vi "Continuous Voltage Ouput - NI.vi"() -> ()   [LabVIEW 2022 SP3]
uses:
  WhiteNoise.ctl
  <vilib>/Utility/error.llb/DialogType.ctl
  <vilib>/DAQmx/write.llb/DAQmx Write (Analog 1D Wfm NChan NSamp).vi
  <vilib>/DAQmx/create/channels.llb/DAQmx Create Channel (AO-Voltage-Basic).vi
  <vilib>/DAQmx/configure/timing.llb/DAQmx Timing (Sample Clock).vi
  <vilib>/measure/maspectr.llb/FFT Spectrum (Mag-Phase) for N Chan.vi
  <vilib>/DAQmx/miscellaneous.llb/DAQmx Fill In Error Info.vi
  <resource>/objmgr/daqmx.rc
  <vilib>/measure/NI_MAPro.lvlib
  <vilib>/measure/NI_MABase.lvlib
panel:
  out "Mag":cluster{"f0":dbl, "df":dbl, "magnitude":dbl[]}[](graph)
  out "Phase":cluster{"f0":dbl, "df":dbl, "phase":dbl[]}[](graph)
  in  "Number of Samples":i32=40000
  in  "Sample Rate":dbl=41200.0
  in  "Sample Clock Source":tag="OnboardClock"
  in  "Max Voltage":dbl=3.5
  in  "Min Voltage":dbl=-3.0
  in  "Physical Channel(s)":tag="Dev1/ao0"
  in  "?":enum32{"White Noise", "Harmonic"}(tab)
  in  "Cluster":T2={"Seed"=0.0, "Standard Deviation"=0.2, "Reset"=FALSE, "Iterator"=1.0} {"Standard Deviation" format="%0.2p"}
  in  "Cluster 2":T3={"Iterator"=1.0, "Waveform Type"=0, "Frequency"=10.0, "Amplitude"=0.5} {"Frequency" format="%0.2p"; "Waveform Type" items=["Sine Wave", "Triangle Wave", "Square Wave", "Sawtooth Wave"]; "Amplitude" format="%0.2p"}
  out "Actual Sample Rate":dbl=1000.0 format="%0.2f"
  in  "Stop":bool
  out "Waveform Graph":waveform(dbl)[](graph)=[{"t0"=timestamp(0 s since 1904-01-01), "dt"=0.001, "Y"=[]}]
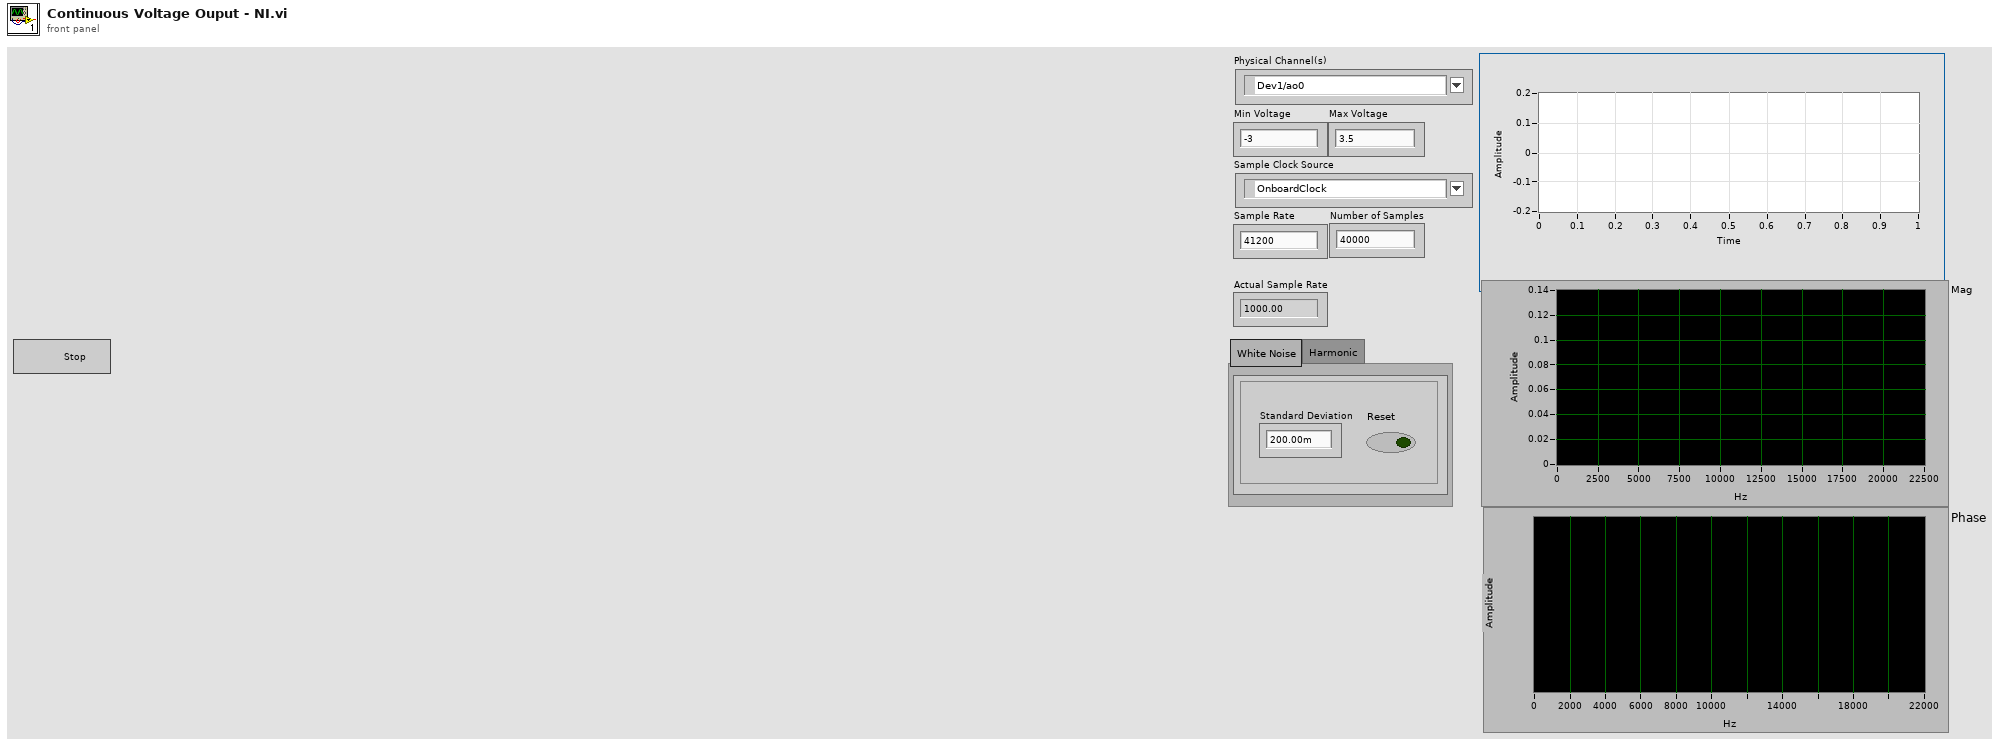
[diagram p1: front panel]
types:
  T1 = typedef "WhiteNoise.ctl" = dbl
  T2 = cluster{"Seed":T1, "Standard Deviation":dbl, "Reset":bool, "Iterator":dbl}
  T3 = cluster{"Iterator":dbl, "Waveform Type":u16, "Frequency":dbl, "Amplitude":dbl}
  T4 = typedef "DialogType.ctl" = u16
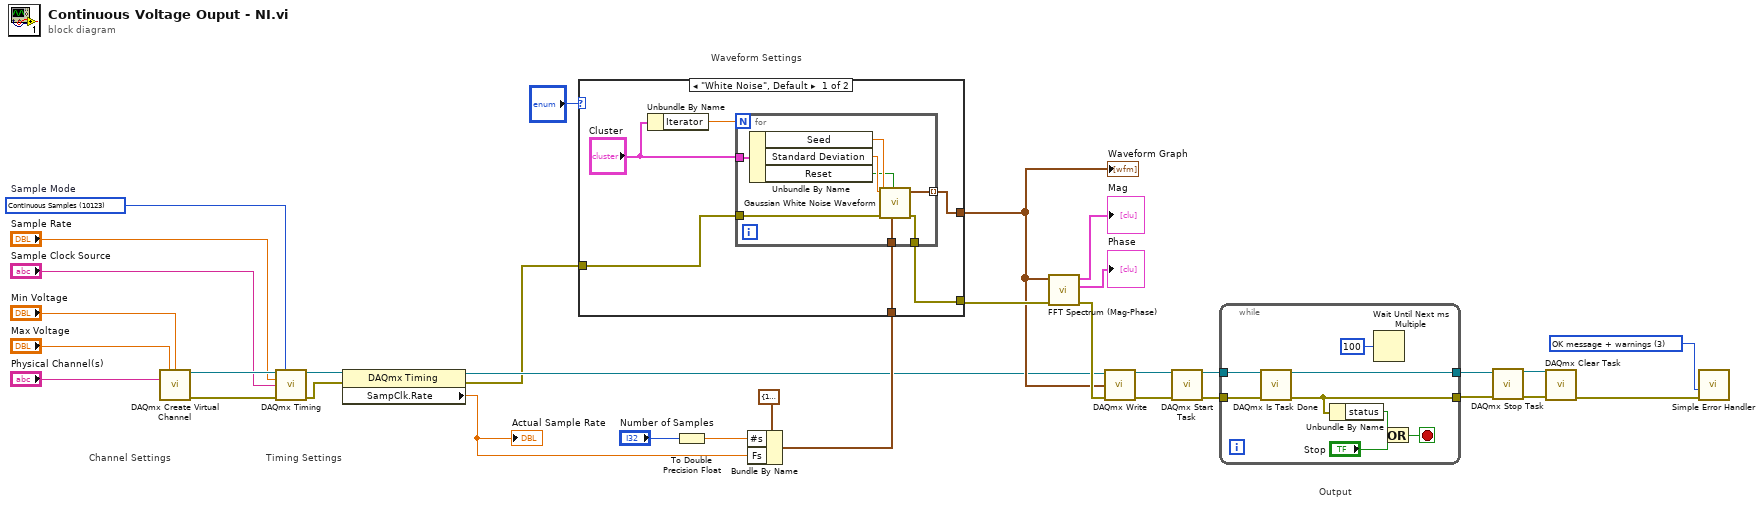
[diagram p0: block diagram]
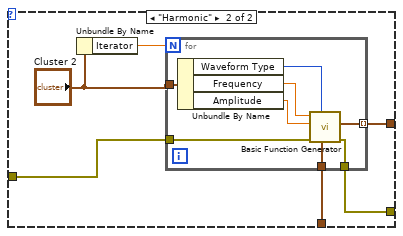
[diagram p2: hidden frame]
diagram:
  w10 = T4 3 items=["no dialog", "OK message", "continue or stop message", "OK message + warnings", "continue/stop + warnings"] ("type of dialog (OK msg:1)")
  w31 = 10123 items=["Finite Samples"=10178, "Continuous Samples"=10123, "Hardware Timed Single Point"=12522]  # Sample Mode
  # "Output"
  # "Waveform Settings"
  # "Timing Settings"
  # "Channel Settings"
  n1 = call-poly <vilib>:"DAQmx Create Virtual Channel.vi"("maximum value"="Max Voltage", "minimum value"="Min Voltage", "physical channels"="Physical Channel(s)") -> ("task out"=w29:refnum<k21>, "error out"=w30:errorcluster)  [unwired: 11 in]
  n2 = call-poly <vilib>:"DAQmx Timing.vi"("task/channels in"=w29, "sample mode"=w31, "rate"="Sample Rate", "source"="Sample Clock Source", "error in"=w30) -> ("task out"=w33:refnum<k21>, "error out"=w32:errorcluster)  [unwired: 9 in]
  n3 = property class="DAQmx Timing"(reference=w33, error in=w32) -> (reference out=w2:refnum<k21>, error out=w1:errorcluster, "SampClk.Rate"=w19:dbl)
  "Actual Sample Rate" <- w19
  n4 = To Double Precision Float(number="Number of Samples") -> (double precision float=w16:dbl)
  n5 = Bundle By Name(cluster=cluster{"Fs":dbl, "#s":dbl} {"Fs"=1000.0, "#s"=1000.0} ("sampling info"), "#s"=w16, "Fs"=w19) -> (w18:cluster{"Fs":dbl, "#s":dbl})
  n6 = case shown="\"White Noise\", Default" "?" {
    tunnel: w18 -> [w39 w51]
    tunnel: w1 -> [w34 w53]
    tunnel: [w38 w50] -> w5
    tunnel: [w35 w52] -> w4
    frame "White Noise", Default {
      n7 = Unbundle By Name("Cluster") -> ("Iterator"=w37:dbl)
      n8 = for {
        N: w37 -> [_]
        tunnel: w34 -> [w47]
        tunnel: w39 -> [w46]
        tunnel: [w45] -> w38
        tunnel: "Cluster" -> [w44]
        tunnel: [w43] -> w35 mode=indexing
        n9 = Unbundle By Name(w44) -> ("Seed"=w42:T1, "Standard Deviation"=w41:dbl, "Reset"=w40:bool)
        n10 = call <vilib>:"Gaussian White Noise Waveform.vi"("sampling info"=w46, "reset signal"=w40, "error in (no error)"=w47, "seed"=w42, "standard deviation"=w41) -> ("error out"=w45:errorcluster, "signal out"=w43:waveform(dbl))  [unwired: 5 in]
      }
    }
    frame "Harmonic" {
      n11 = Unbundle By Name("Cluster 2") -> ("Iterator"=w49:dbl)
      n12 = for {
        N: w49 -> [_]
        tunnel: w53 -> [w61]
        tunnel: w51 -> [w60]
        tunnel: [w59] -> w50
        tunnel: "Cluster 2" -> [w58]
        tunnel: [w54] -> w52 mode=indexing
        n13 = Unbundle By Name(w58) -> ("Waveform Type"=w57:u16, "Frequency"=w56:dbl, "Amplitude"=w55:dbl)
        n14 = call <vilib>:"Basic Function Generator.vi"("sampling info"=w60, "signal type"=w57, "error in (no error)"=w61, "amplitude"=w55, "frequency"=w56) -> ("error out"=w59:errorcluster, "signal out"=w54:waveform(dbl))  [unwired: 4 in, 1 out]
      }
    }
  }
  "Waveform Graph" <- w4
  n15 = call-poly <vilib>:"FFT Spectrum (Mag-Phase).vi"("error in (no error)"=w5, "time signals"=w4) -> ("error out"=w6:errorcluster, "phases"=→"Phase":cluster{"f0":dbl, "df":dbl, "phase":dbl[]}[], "magnitudes"=→"Mag":cluster{"f0":dbl, "df":dbl, "magnitude":dbl[]}[])  [unwired: 5 in, 2 out]
  n16 = call-poly <vilib>:"DAQmx Write.vi"("task/channels in"=w2, "data"=w4, "error in"=w6) -> ("task out"=w17:refnum<k21>, "error out"=w9:errorcluster)  [unwired: 10 in, 1 out]
  n17 = call <vilib>:"DAQmx Start Task.vi"("task/channels in"=w17, "error in"=w9) -> ("task out"=w28:refnum<k21>, "error out"=w27:errorcluster)  [unwired: 12 in]
  n18 = while {
    tunnel: w28 -> [w69]
    tunnel: w27 -> [w68]
    tunnel: [w65] -> w11
    tunnel: [w66] -> w12
    stop <- w67 stop-if-true
    n19 = call <vilib>:"DAQmx Is Task Done.vi"("task/channels in"=w69, "error in"=w68) -> ("task out"=w66:refnum<k21>, "error out"=w65:errorcluster)  [unwired: 11 in, 1 out]
    n20 = Unbundle By Name(w65) -> ("status"=w64:bool)
    n21 = Wait Until Next ms Multiple(millisecond multiple=u32 100) -> ()  [unwired: 1 out]
    n22 = Or(x=w64, y="Stop") -> (x .or. y?=w67:bool)
  }
  n23 = call <vilib>:"DAQmx Stop Task.vi"("task/channels in"=w12, "error in"=w11) -> ("task out"=w14:refnum<k21>, "error out"=w13:errorcluster)  [unwired: 12 in]
  n24 = call <vilib>:"DAQmx Clear Task.vi"("task in"=w14, "error in"=w13) -> ("error out"=w26:errorcluster)  [unwired: 13 in]
  n25 = call <vilib>:"Simple Error Handler.vi"("type of dialog (OK msg:1)"=w10, "error in (no error)"=w26) -> ()  [unwired: 3 in, 5 out]
